vi "Byte Buffer.Resize.vi"(8 "error in (no error)":errorcluster, 10 "new size":u64, 11 "Byte Buffer in":refnum<class "Byte Buffer.lvclass">) -> (0 "error out":errorcluster, 3 "Byte Buffer out":refnum<class "Byte Buffer.lvclass">)   [LabVIEW 2016, in "VeriStand Data.lvlib" / "Byte Buffer.lvclass"]
doc: "Resizes the provided <B>buffer</B>, preserving the current contents of the buffer. If the <B>new size</B> is smaller than the previous size, the buffered data beyond the new buffer size is discarded."
uses:
  Byte Buffer.lvclass
  Byte Buffer.lvclass/Byte Buffer.ctl
  Memory Management/Memory Management.Handle Return.vi
  VeriStand Data.lvlib
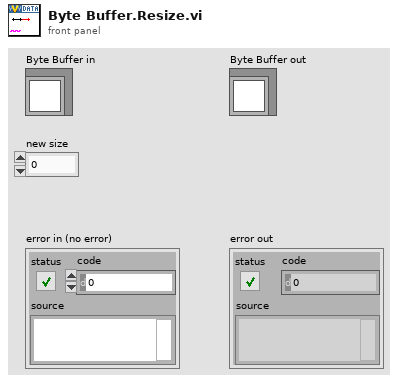
[diagram p1: front panel]
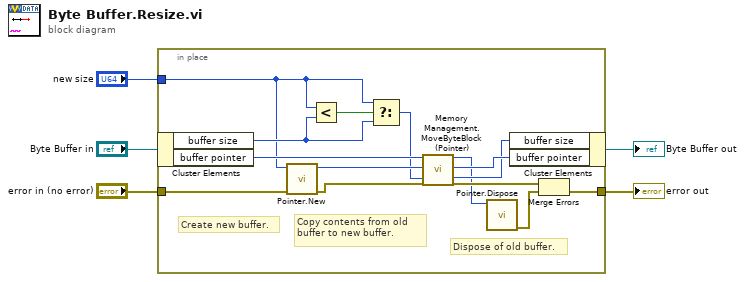
[diagram p0: block diagram]
diagram:
  n1 = in-place {
    in-place-border: "error in (no error)" -> [w15]
    in-place-border: "new size" -> [w11]
    in-place-border: [w8] -> w1
    # "Dispose of old buffer."
    # "Copy contents from old buffer to new buffer."
    # "Create new buffer."
    n2 = in-place-cluster #1("Byte Buffer in") -> ("buffer size"=w12:u64, "buffer pointer"=w16:u64)
    n3 = call "Pointer.New.vi"("error in (no error)"=w15, "size in bytes"=w11) -> ("error out"=w19:errorcluster, "pointer"=w18:u64)  [unwired: 8 in]
    n4 = Less?(x=w11, y=w12) -> (x < y?=w17:bool)
    n5 = Select(t=w11, s=w17, f=w12) -> (s? t:f=w13:u64)
    n6 = call "Memory Management.MoveByteBlock (Pointer).vi"("src ptr in"=w16, "dst ptr in"=w18, "size"=w13, "error in (no error)"=w19) -> ("src ptr out"=w6:u64, "dst ptr out"=w14:u64, "size out"=w7:u64, "error out"=w10:errorcluster)  [unwired: 10 in, 2 out]
    n7 = call "Pointer.Dispose.vi"("pointer"=w6) -> ("error out"=w9:errorcluster)  [unwired: 9 in, 1 out]
    n8 = in-place-cluster #1("buffer size"=w7, "buffer pointer"=w14) -> (→"Byte Buffer out":refnum<class "Byte Buffer.lvclass">)
    n9 = Merge Errors(w10, w9) -> (w8:errorcluster)
  }
  "error out" <- w1
